vi "FromClusterToTagBusScript.vi"(5 "process":T1={"param?"=TRUE, "Parameter Data Interface VI (blank=tag bus to parameters.vi)"="", "Result Data Interface VI (blank=results to tag bus.vi)"="", "reverse param?"=FALSE, "Rev. Result Interface VI (blank=results from tag bus.vi)"="", "Rev. Parameter Interface VI (blank=tag bus from parameters.vi)"="", "result?"=TRUE, "reverse result?"=FALSE}, 7 "output":T2={"enable?"=TRUE, "Data Interface VI (blank=tag bus to outputs.vi)"="", "Reverse Interface VI (blank=tag bus from outputs.vi)"="", "reverse?"=FALSE}, 8 "error in":errorcluster, 10 "input":T3={"enable?"=TRUE, "Data Interface VI (blank=input to tag bus.vi)"="", "reverse?"=FALSE, "Reverse Interface VI (blank=input from tag bus.vi)"=""}, 11 "runtime class path":path) -> (0 "error out":errorcluster)   [LabVIEW 2013, in "data interface script.lvlib"]
doc: "THis Vi scripts the index cluster and the VI to convert from a cluster into Tagbus"
uses:
  data interface script.lvlib
  Controls/input script control.ctl
  Controls/output script control.ctl
  Controls/processing script control.ctl
  Controls/ControlsProperties.ctl
  <vilib>/Utility/miscctls.llb/LVPointTypeDef.ctl
  Controls/StateCluster.ctl
  Controls/initialized references.ctl
  Controls/interface VI type.ctl
panel:
  in  "configuration class path":path
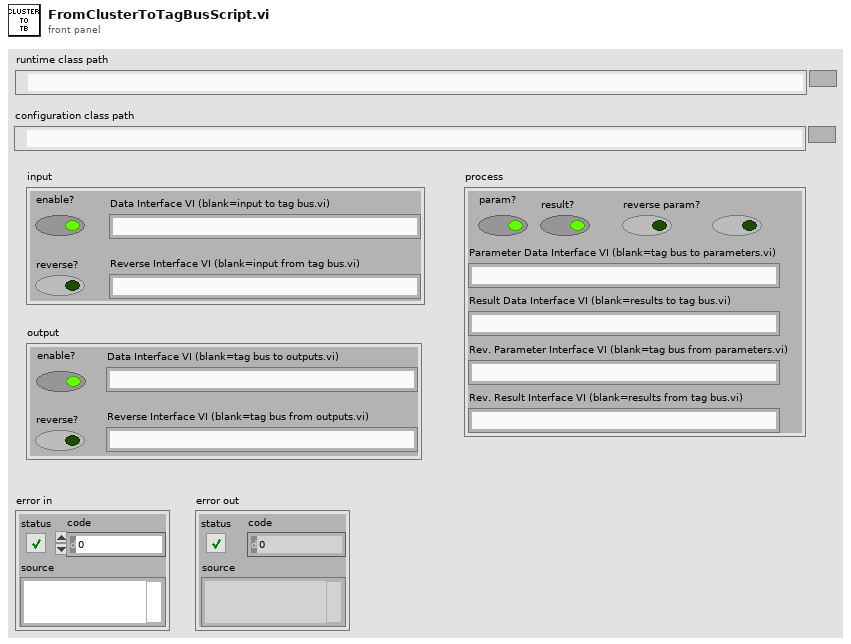
[diagram p1: front panel]
types:
  T1 = typedef "data interface script.lvlib/processing script control.ctl" = cluster{"param?":bool, "Parameter Data Interface VI (blank=tag bus to parameters.vi)":string, "Result Data Interface VI (blank=results to tag bus.vi)":string, "reverse param?":bool, "Rev. Result Interface VI (blank=results from tag bus.vi)":string, "Rev. Parameter Interface VI (blank=tag bus from parameters.vi)":string, "result?":bool, "reverse result?":bool}
  T2 = typedef "data interface script.lvlib/output script control.ctl" = cluster{"enable?":bool, "Data Interface VI (blank=tag bus to outputs.vi)":string, "Reverse Interface VI (blank=tag bus from outputs.vi)":string, "reverse?":bool}
  T3 = typedef "data interface script.lvlib/input script control.ctl" = cluster{"enable?":bool, "Data Interface VI (blank=input to tag bus.vi)":string, "reverse?":bool, "Reverse Interface VI (blank=input from tag bus.vi)":string}
  T4 = typedef "data interface script.lvlib/ControlsProperties.ctl" = cluster{"label":string, "terminal index":u32, "indicator":bool, "location":T5}
  T5 = typedef "LVPointTypeDef.ctl" = cluster{"Horizontal":i16, "Vertical":i16}
  T6 = typedef "data interface script.lvlib/initialized references.ctl" = cluster{"data ctl":refnum<vi>, "index ctl":refnum<vi>, "interface vi":refnum<vi>, "vi type":T7}
  T7 = typedef "data interface script.lvlib/interface VI type.ctl" = enum16{"tb to data", "data to tb"}
  T8 = typedef "data interface script.lvlib/StateCluster.ctl" = cluster{"base cluster":variant, "vi refs":T6}
  T9 = typedef "data interface script.lvlib/TerminalReferences.ctl" = cluster{"Cluster":refnum<vi>, "Index Cluster":refnum<vi>, "tag bus in":refnum<vi>, "tag bus out":refnum<vi>}
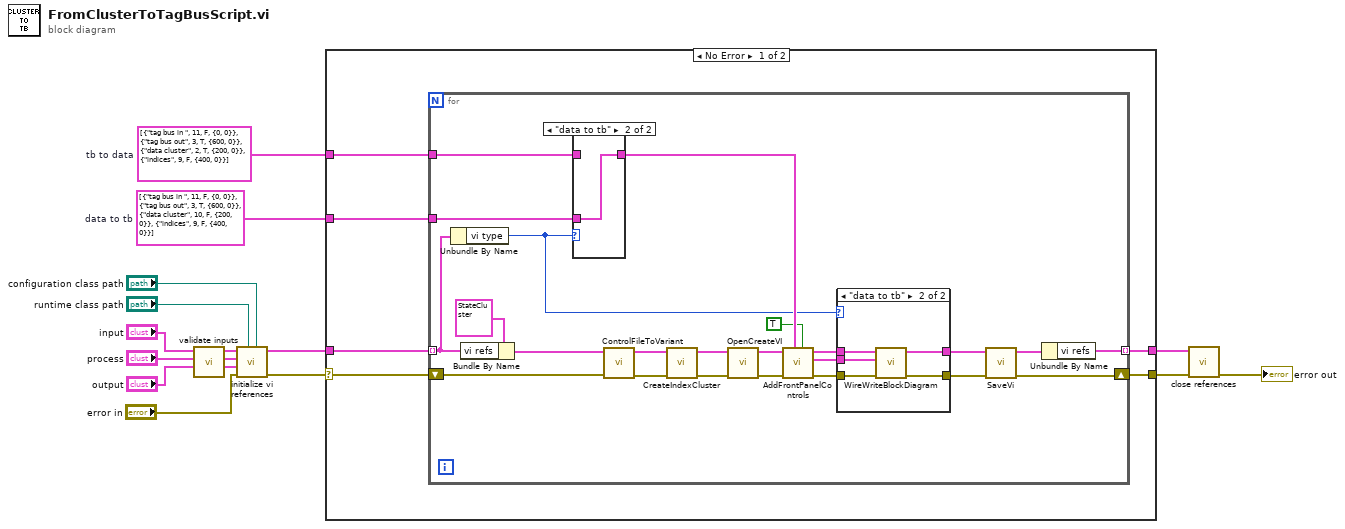
[diagram p0: block diagram]
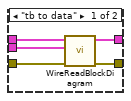
[diagram p2: hidden frame]
diagram:
  w2 = T4[] [{"label"="tag bus in ", "terminal index"=11, "indicator"=FALSE, "location"={"Horizontal"=0, "Vertical"=0}}, {"label"="tag bus out", "terminal index"=3, "indicator"=TRUE, "location"={"Horizontal"=600, "Vertical"=0}}, {"label"="data cluster", "terminal index"=10, "indicator"=FALSE, "location"={"Horizontal"=200, "Vertical"=0}}, {"label"="indices", "terminal index"=9, "indicator"=FALSE, "location"={"Horizontal"=400, "Vertical"=0}}]  # data to tb
  w3 = T4[] [{"label"="tag bus in ", "terminal index"=11, "indicator"=FALSE, "location"={"Horizontal"=0, "Vertical"=0}}, {"label"="tag bus out", "terminal index"=3, "indicator"=TRUE, "location"={"Horizontal"=600, "Vertical"=0}}, {"label"="data cluster", "terminal index"=2, "indicator"=TRUE, "location"={"Horizontal"=200, "Vertical"=0}}, {"label"="indices", "terminal index"=9, "indicator"=FALSE, "location"={"Horizontal"=400, "Vertical"=0}}]  # tb to data
  n1 = call "validate inputs.vi"("output in"="output", "process in"="process", "input in"="input") -> ("output out"=w11:T2, "process out"=w12:T1, "input out"=w13:T3)  [unwired: 6 in]
  n2 = call "initialize vi references.vi"("config class path"="configuration class path", "runtime class path"="runtime class path", "error in"="error in", "output in"=w11, "process in"=w12, "input in"=w13) -> ("error out"=w9:errorcluster, "initialized references"=w8:T6[])  [unwired: 4 in]
  n3 = case shown="No Error" w9 {
    selector: w9 -> [w21 w59]
    tunnel: w8 -> [w22 w58]
    tunnel: [w20 w59] -> w5
    tunnel: [w17 w58] -> w6
    tunnel: w3 -> [w19 _]
    tunnel: w2 -> [w18 _]
    frame No Error {
      n4 = for {
        tunnel: w22 -> [w42] mode=indexing
        shift-right: [w25] -> w20
        shift-left: w21 -> [w40]
        tunnel: w19 -> [w45]
        tunnel: w18 -> [w44]
        tunnel: [w23] -> w17 mode=indexing
        n5 = Unbundle By Name(w42) -> ("vi type"=w31:T7)
        n6 = Bundle By Name(cluster=T8 {"base cluster"=variant, "vi refs"={"data ctl"=refnum, "index ctl"=refnum, "interface vi"=refnum, "vi type"=enum."tb to data"}} ("State"), "vi refs"=w42) -> (w41:T8)
        n7 = case shown="\"data to tb\"" w31 {
          tunnel: [w56 w57] -> w33
          tunnel: w45 -> [w56 _]
          tunnel: w44 -> [_ w57]
          frame "tb to data" {
          }
          frame "data to tb" {
          }
        }
        n8 = call "ControlFileToVariant.vi"("error in"=w40, "State"=w41) -> ("error out"=w38:errorcluster, "State out"=w39:T8)  [unwired: 8 in]
        n9 = call "CreateIndexCluster.vi"("error in"=w38, "State"=w39) -> ("error out"=w36:errorcluster, "State out"=w37:T8)  [unwired: 8 in]
        n10 = call "OpenCreateVI.vi"("error in"=w36, "State"=w37) -> ("error out"=w35:errorcluster, "State out"=w34:T8)  [unwired: 8 in]
        n11 = call "AddFrontPanelControls.vi"("Open Front Panel"=TRUE, "Control Properties"=w33, "error in"=w35, "State"=w34) -> ("error out"=w28:errorcluster, "Terminal References"=w29:T9, "State out"=w30:T8)  [unwired: 5 in]
        n12 = case shown="\"data to tb\"" w31 {
          tunnel: w30 -> [w50 w55]
          tunnel: w29 -> [w49 w54]
          tunnel: w28 -> [w48 w53]
          tunnel: [w47 w52] -> w26
          tunnel: [w46 w51] -> w27
          frame "tb to data" {
            n13 = call "WireReadBlockDiagram.vi"("error in"=w48, "Terminal References"=w49, "State"=w50) -> ("error out"=w47:errorcluster, "State out"=w46:T8)  [unwired: 7 in]
          }
          frame "data to tb" {
            n14 = call "WireWriteBlockDiagram.vi"("error in"=w53, "Terminal References"=w54, "State"=w55) -> ("error out"=w52:errorcluster, "State out"=w51:T8)  [unwired: 7 in]
          }
        }
        n15 = call "SaveVi.vi"("error in"=w26, "State"=w27) -> ("error out"=w25:errorcluster, "State out"=w24:T8)  [unwired: 8 in]
        n16 = Unbundle By Name(w24) -> ("vi refs"=w23:T6)
      }
    }
    frame Error {
    }
  }
  n17 = call "close references.vi"("error in"=w5, "initialized references"=w6) -> ("error out"=→"error out":errorcluster)  [unwired: 9 in]
